vi "Get Current Waveform.vi"(9 "Config":T1={"Channel Index"=1, "Resistance"=2, "Channel name"="Source-Current"}, 11 "array":waveform(dbl)[](array[waveform])) -> (1 "Channel name":string, 3 "waveform out":waveform(dbl))   [LabVIEW 2019]
doc: "This example demonstrates how to acquire a continuous amount of data (Waveform) using the DAQ device's internal clock. It also shows how to synchronize two devices for different device families (E Series, S Series, M Series, X Series, DSA, and SC Express), to simultaneously acquire the data.\n\nFor instructions on how to connect your signals to the DAQ device, refer to your device documentation."
panel:
  # "Get Current Waveform"
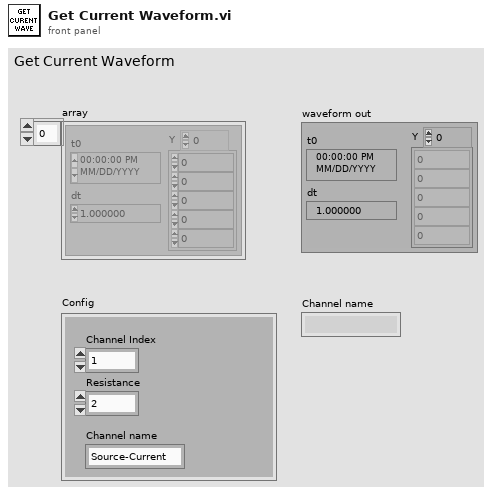
[diagram p1: front panel]
types:
  T1 = cluster{"Channel Index":i32, "Resistance":i32, "Channel name":string}
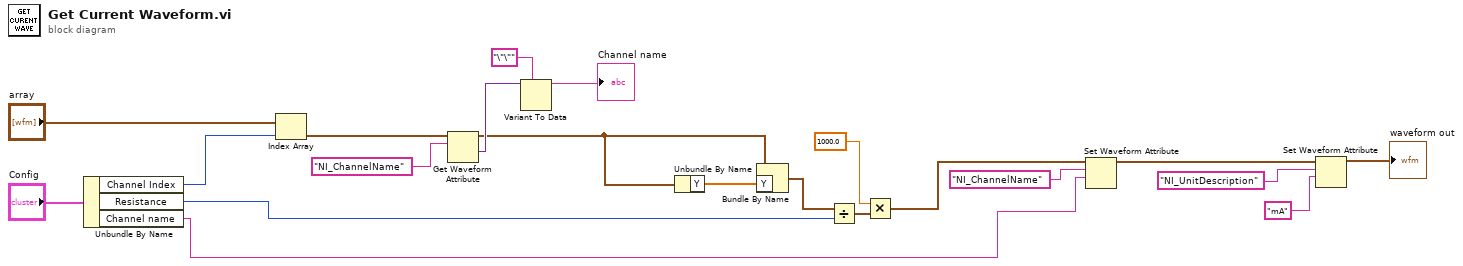
[diagram p0: block diagram]
diagram:
  n1 = Unbundle By Name("Config") -> ("Channel Index"=w12:i32, "Resistance"=w6:i32, "Channel name"=w4:string)
  n2 = Index Array(array="array", index=w12) -> (element=w16:waveform(dbl))
  n3 = Get Waveform Attribute(6:"NI_ChannelName" ("name"), 7:w16) -> (1:w10:variant, 3:w7:waveform(dbl))  [unwired: 2 in, 2 out]
  n4 = Variant To Data(type="\"\"" ("name"), Variant=w10) -> (data=→"Channel name":string)  [unwired: 1 in, 1 out]
  n5 = Unbundle By Name(w7) -> ("Y"=w5:dbl[])
  n6 = Bundle By Name(cluster=w7, "Y"=w5) -> (w8:waveform(dbl))
  n7 = Divide(x=w8, y=w6) -> (x/y=w3:waveform(dbl))
  n8 = Multiply(x=1000.0, y=w3) -> (x*y=w2:waveform(dbl))
  n9 = Set Waveform Attribute(5:w4, 6:"NI_ChannelName" ("name"), 7:w2) -> (3:w18:waveform(dbl))  [unwired: 1 in, 2 out]
  n10 = Set Waveform Attribute(5:"mA" ("name"), 6:"NI_UnitDescription" ("name"), 7:w18) -> (3:→"waveform out":waveform(dbl))  [unwired: 1 in, 2 out]
